vi "QMH Template.vi"() -> ()   [LabVIEW 2009, in "AMC Templates.lvlib"]
uses:
  AMC Templates.lvlib
  AMC.lvlib
panel:
  out "status":string
  in  "process":bool
  in  "exit":bool
  in  "state variables":cluster{"CurrentFile":path}
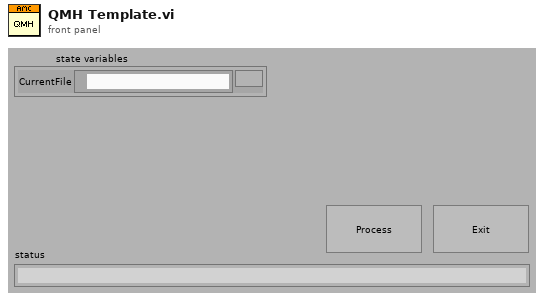
[diagram p1: front panel]
types:
  T1 = typedef "AMC.lvlib/Message Queue.ctl" = refnum<queue>
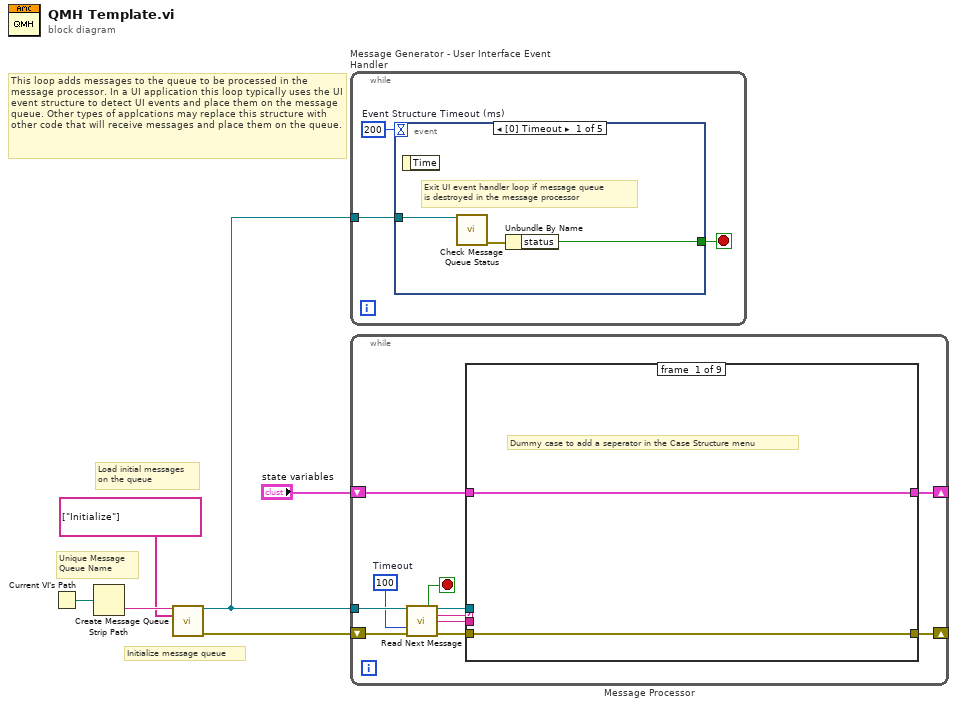
[diagram p0: block diagram]
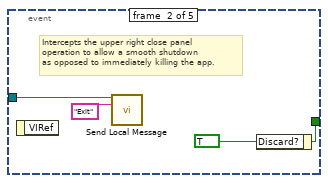
[diagram p2: hidden frame]
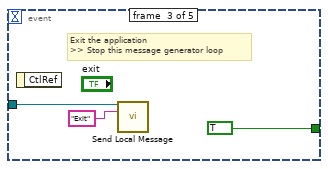
[diagram p3: hidden frame]
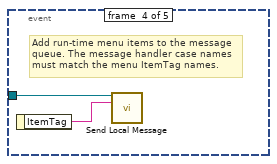
[diagram p4: hidden frame]
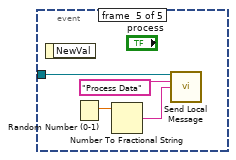
[diagram p5: hidden frame]
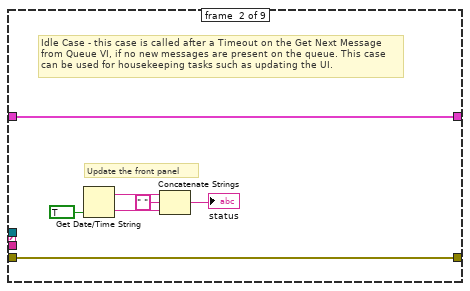
[diagram p6: hidden frame]
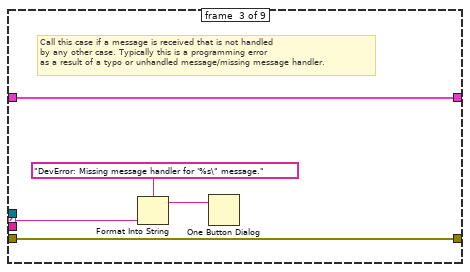
[diagram p7: hidden frame]
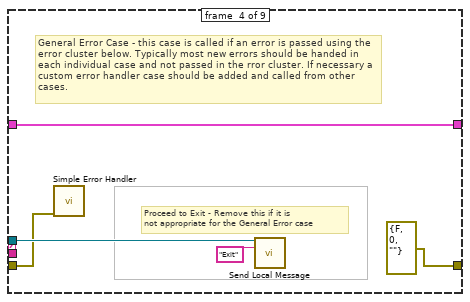
[diagram p8: hidden frame]
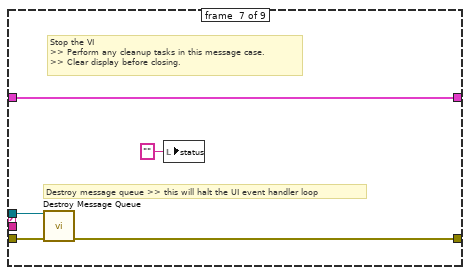
[diagram p11: hidden frame]
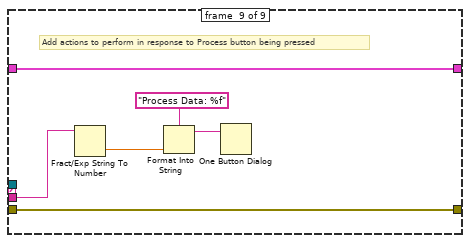
[diagram p13: hidden frame]
diagram:
  # "This loop adds messages to the queue to be processed in the message processor. In a UI application this loop typically uses the UI event structure to detect UI events and place them on the message queue. Other types of applcations may replace this structure with other code that will receive messages and place them on the queue."
  # "Initialize message queue"
  # "Unique Message\nQueue Name"
  # "Load initial messages\non the queue"
  n1 = Current VI's Path() -> (path=w6:path)
  n2 = Strip Path(path=w6) -> (name=w2:string)  [unwired: 1 out]
  n3 = call "Create Message Queue.vi"("message queue name"=w2, "initial message names"=string[] ["Initialize"]) -> ("message queue out"=w3:T1, "error out"=w4:errorcluster)  [unwired: 12 in]
  n4 = while "Message Generator - User Interface Event Handler" {
    tunnel: w3 -> [w7]
    stop <- w8 stop-if-true
    w9 = 200  # Event Structure Timeout (ms)
    n5 = event shown="[0] Timeout" {
      selector: _ -> [_ _ _ _ _]
      dyn-events: _ -> [_ _ _ _ _]
      timeout: w9 -> [_ _ _ _ _]
      tunnel: [w10 w15 TRUE ("Discard?") _ _] -> w8
      tunnel: w7 -> [w11 w13 w16 w19 w24]
      event #0 {
        # "Exit UI event handler loop if message queue\nis destroyed in the message processor"
        n6 = event-data() -> ()  [unwired: 2 out]
        n7 = call "Check Message Queue Status.vi"("message queue in"=w11) -> ("error out"=w12:errorcluster)  [unwired: 10 in, 4 out]
        n8 = Unbundle By Name(w12) -> ("status"=w10:bool)
      }
      event #1 {
        w15 = TRUE ("Discard?")
        # "Intercepts the upper right close panel\noperation to allow a smooth shutdown\nas opposed to immediately killing the app."
        n9 = event-data() -> ()  [unwired: 2 out]
        n10 = call "Send Local Message.vi"("message queue in"=w13, "message name"="Exit") -> ()  [unwired: 11 in, 3 out]
        n11 = event-data("Discard?"=w15) -> ()  [unwired: 1 in, 1 out]
      }
      event #2 {
        # "Exit the application\n>> Stop this message generator loop"
        n12 = event-data() -> ()  [unwired: 2 out]
        n13 = call "Send Local Message.vi"("message queue in"=w16, "message name"="Exit") -> ()  [unwired: 11 in, 3 out]
      }
      event #3 {
        # "Add run-time menu items to the message\nqueue. The message handler case names must match the menu ItemTag names."
        n14 = event-data() -> ("ItemTag"=w20:string)  [unwired: 1 out]
        n15 = call "Send Local Message.vi"("message queue in"=w19, "message name"=w20) -> ()  [unwired: 11 in, 3 out]
      }
      event #4 {
        n16 = event-data() -> ()  [unwired: 2 out]
        n17 = Random Number (0-1)() -> (number: 0 to 1=w21:dbl)
        n18 = Number To Fractional String(number=w21) -> (F-format string=w22:string)  [unwired: 3 out]
        n19 = call "Send Local Message.vi"("message queue in"=w24, "message name"="Process Data", "message value"=w22) -> ()  [unwired: 10 in, 3 out]
      }
    }
  }
  n20 = while "Message Processor" {
    shift-left: w4 -> [w29]
    shift-right: [w33] -> _
    tunnel: w3 -> [w30]
    shift-left: "state variables" -> [w35]
    shift-right: [w34] -> _
    stop <- w32 stop-if-true
    w25 = 100  # Timeout
    n21 = call "Read Next Message.vi"("message queue in"=w30, "timeout (1 ms)"=w25, "error in"=w29) -> ("exit process?"=w32:bool, "message queue out"=w31:T1, "message name"=w27:string, "message value"=w26:string, "error out"=w28:errorcluster)  [unwired: 5 in, 3 out]
    n22 = case shown="\"\", \"Idle\"" w27 {
      selector: w27 -> [_ _ w47 _ _ _ _ _ _]
      tunnel: [w37 w44 w49 w54 w56 w58 w63 w65 w70] -> w34
      tunnel: w35 -> [w37 w44 w49 w54 w56 w58 w63 w65 w70]
      tunnel: w31 -> [_ _ _ w52 _ _ w60 _ _]
      tunnel: w28 -> [w36 w43 w48 w50 w55 w57 w61 w64 w71]
      tunnel: [w36 w43 w48 errorcluster {"status"=FALSE, "code"=0, "source"=""} ("error out") w55 w57 w59 w64 w71] -> w33
      tunnel: w26 -> [_ _ _ _ _ _ _ _ w69]
      frame #0 {
        # "Dummy case to add a seperator in the Case Structure menu"
      }
      frame #1 {
        # "Update the front panel"
        # "Idle Case - this case is called after a Timeout on the Get Next Message from Queue VI, if no new messages are present on the queue. This case can be used for housekeeping tasks such as updating the UI."
        n23 = Get Date/Time String(want seconds? (F)=TRUE) -> (date string=w42:string, time string=w41:string)  [unwired: 2 out]
        n24 = Concatenate Strings(w42, " " ("string"), w41) -> (→"status":string)
      }
      frame #2 {
        # "Call this case if a message is received that is not handled \nby any other case. Typically this is a programming error\nas a result of a typo or unhandled message/missing message handler."
        n25 = Format Into String(format string="DevError: Missing message handler for '%s\" message." ("message"), w47) -> (resulting string=w45:string)  [unwired: 2 in, 1 out]
        n26 = One Button Dialog(message=w45) -> ()  [unwired: 2 out]
      }
      frame #3 {
        # "Proceed to Exit - Remove this if it is\nnot appropriate for the General Error case"
        # "General Error Case - this case is called if an error is passed using the error cluster below. Typically most new errors should be handed in each individual case and not passed in the rror cluster. If necessary a custom error handler case should be added and called from other cases."
        n27 = call <vilib>:"Simple Error Handler.vi"("error in (no error)"=w50) -> ()  [unwired: 1 in, 8 out]
        n28 = call "Send Local Message.vi"("message queue in"=w52, "message name"="Exit") -> ()  [unwired: 11 in, 3 out]
      }
      frame #4 {
        # "Dummy case to add a seperator in the Case Structure menu"
      }
      frame #5 {
        # "Initialize the state variables and user interface"
      }
      frame #6 {
        # "Destroy message queue >> this will halt the UI event handler loop"
        # "Stop the VI\n>> Perform any cleanup tasks in this message case.\n>> Clear display before closing."
        n29 = call "Destroy Message Queue.vi"("message queue in"=w60, "error in"=w61) -> ("error out"=w59:errorcluster)  [unwired: 11 in, 2 out]
        n30 = local write "status"("" ("Status")) -> ()
      }
      frame #7 {
        # "Dummy case to add a seperator in the Case Structure menu"
      }
      frame #8 {
        # "Add actions to perform in response to Process button being pressed"
        n31 = Fract/Exp String To Number(string=w69) -> (number=w68:dbl)  [unwired: 4 out]
        n32 = Format Into String(format string="Process Data: %f" ("message"), w68) -> (resulting string=w66:string)  [unwired: 2 in, 1 out]
        n33 = One Button Dialog(message=w66) -> ()  [unwired: 2 out]
      }
    }
  }
